vi "GetCalsFromFile.vi"() -> ()   [LabVIEW 2019]
uses:
  <vilib>/Utility/file.llb/Read Delimited Spreadsheet (string).vi
  <vilib>/Rock Robotics/Network Tables/NT Write String Array.vi
panel:
  in  "Enum 2":T1(ring)
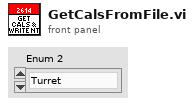
[diagram p1: front panel]
types:
  T1 = enum16{"Turret", "Magazine", "Intake", "Flywheel", "Drive", "Climb", "Control_Panel_"}
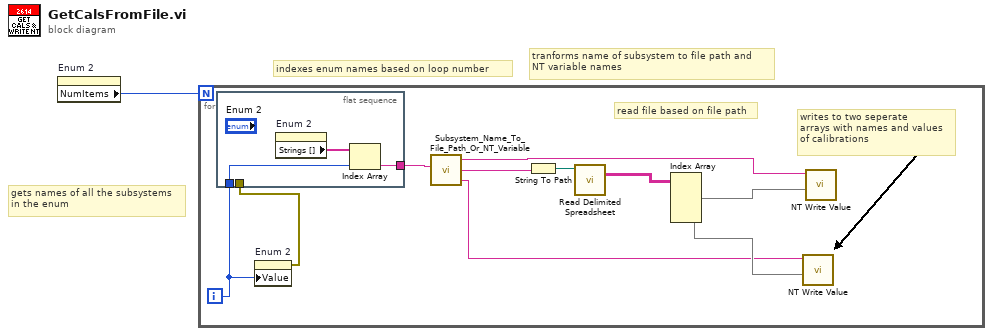
[diagram p0: block diagram]
diagram:
  # "tranforms name of subsystem to file path and\nNT variable names"
  # "indexes enum names based on loop number"
  # "gets names of all the subsystems\nin the enum"
  n1 = property on="Enum 2" class="Enum (strict)"() -> ("NumItems"=w1:u32)  [unwired: 2 in, 2 out]
  n2 = for {
    N: w1 -> [_]
    i -> [w3]
    # "writes to two seperate\narrays with names and values\nof calibrations"
    # "read file based on file path"
    n3 = flat-sequence {
      tunnel: w4 -> [_]
      tunnel: w3 -> [w13]
      tunnel: [w12] -> w2
      frame #0 {
        n4 = property on="Enum 2" class="Enum (strict)"() -> ("Strings []"=w14:string[])  [unwired: 2 in, 2 out]
        n5 = Index Array(array=w14, index=w13) -> (element=w12:string)
      }
    }
    n6 = property on="Enum 2" class="Enum (strict)"("Value"=w3) -> (error out=w4:errorcluster)  [unwired: 2 in, 1 out]
    n7 = call "Subsystem_Name_To_File_Path_Or_NT_Variable.vi"("Enum String Name"=w2) -> ("Names"=w6:string, "File Path"=w7:string, "Values"=w5:string)  [unwired: 5 in]
    n8 = String To Path(string=w7) -> (path=w8:path)
    n9 = call-poly <vilib>:"Read Delimited Spreadsheet.vi"("file path (dialog if empty)"=w8) -> ("all rows"=w11:string[][])  [unwired: 9 in, 5 out]
    n10 = Index Array(array=w11) -> (element #1=w9:string[], element #2=w10:string[])  [unwired: 4 in]
    n11 = call-poly <vilib>:"NT Write Value.vi"("String Array"=w10, "Name"=w5) -> ()  [unwired: 9 in, 1 out]
    n12 = call-poly <vilib>:"NT Write Value.vi"("String Array"=w9, "Name"=w6) -> ()  [unwired: 9 in, 1 out]
  }
